vi "Calculate Waveform.vi"(6 "Channel":enum16{"Invalid", "Channel 1", "Channel 2"}(ring), 8 "error in (no error)":errorcluster, 9 "Acquisition Time":timestamp, 10 "Points":i16[](array[numeric]), 11 "OWON SDS1022 in":refnum<class "OWON SDS1022.lvclass">) -> (0 "error out":errorcluster, 3 "OWON SDS1022 out":refnum<class "OWON SDS1022.lvclass">)   [LabVIEW 2023, in "OWON SDS1022.lvclass"]
uses:
  Continuous Waveform Acq CFG.lvclass/Continuous Waveform Acq CFG.ctl
  OWON SDS1022.lvclass
  OWON SDS1022.lvclass/OWON SDS1022.ctl
  5ff70b4c-a951-438e-aa90-247ca6a210be.vi
  <vilib>/Utility/error.llb/Error Cluster From Error Code.vi
  <vilib>/ErrorRing/Error Ring.xnode
  f43ade27-b117-4f32-80ae-6d7f201a5a9d.vi
  7c31662c-ba05-4203-8e23-b7890d435081.vi
  b003ad20-f1c5-4d81-8556-46127c723614.vi
  HAL/Scope Base/Scope Base.lvclass
  E:/git/HAL/Scope VISA/Scope VISA.lvclass
  E:/git/HAL/Scope Base/Scope Base.lvclass
  E:/git/HAL/Hardware_class/Instrument.lvclass
  E:/git/HAL/Interfaces/IScope/IScope.lvclass
  E:/git/OWON-SDS1022-LabVIEW/OWON SDS1022/OWON SDS1022.lvclass
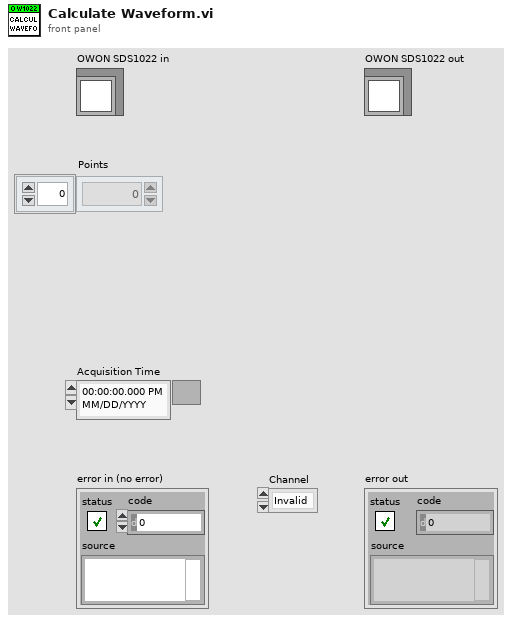
[diagram p1: front panel]
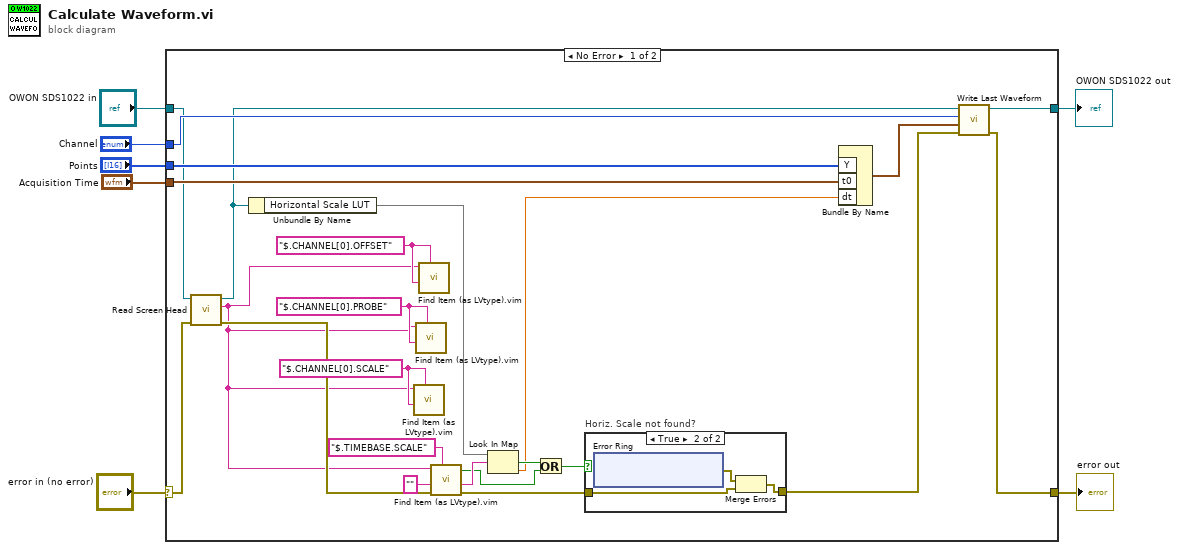
[diagram p0: block diagram]
diagram:
  n1 = case shown="No Error" "error in (no error)" {
    selector: "error in (no error)" -> [w27 w42]
    tunnel: [w14 w42] -> w6
    tunnel: [w13 w41] -> w4
    tunnel: "OWON SDS1022 in" -> [w10 w41]
    tunnel: "Points" -> [w23 _]
    tunnel: "Acquisition Time" -> [w22 _]
    tunnel: "Channel" -> [w12 _]
    frame No Error {
      w17 = "$.CHANNEL[0].OFFSET" ("$Path or Item Name")
      w16 = "$.CHANNEL[0].PROBE" ("$Path or Item Name")
      w15 = "$.CHANNEL[0].SCALE" ("$Path or Item Name")
      n2 = call "Read Screen Head.vi"("error in"=w27, "OWON SDS1022.lvclass"=w10) -> ("error out"=w30:errorcluster, "Head <JSON>"=w9:string, "OWON SDS1022.lvclass 2"=w8:refnum<class "OWON SDS1022.lvclass">)  [unwired: 7 in]
      n3 = Unbundle By Name(w8) -> ("Horizontal Scale LUT"=w19:map{string, dbl})
      n4 = call "Find Item (as LVtype).vim"("$Path or Item Name"=w15, "Data Type and Default Value"=w15, "JSON"=w9) -> ()  [unwired: 5 in, 4 out]
      n5 = call "Find Item (as LVtype).vim"("$Path or Item Name"=w16, "Data Type and Default Value"=w16, "JSON"=w9) -> ()  [unwired: 5 in, 4 out]
      n6 = call "Find Item (as LVtype).vim"("$Path or Item Name"=w17, "Data Type and Default Value"=w17, "JSON"=w9) -> ()  [unwired: 5 in, 4 out]
      n7 = call "Find Item (as LVtype).vim"("$Path or Item Name"="$.TIMEBASE.SCALE", "error in (no error)"=w30, "Data Type and Default Value"="", "JSON"=w9) -> ("error out"=w26:errorcluster, "Data"=w28:string, "Found"=w20:bool)  [unwired: 4 in, 1 out]
      n8 = Look In Map(map=w19, key=w28) -> (key not found?=w24:bool, value=w18:dbl)  [unwired: 1 in]
      n9 = Or(x=w24, y=w20) -> (x .or. y?=w21:bool)
      n10 = case "Horiz. Scale not found?" shown="True" w21 {
        tunnel: w26 -> [w32 w34]
        tunnel: [w32 w33] -> w25
        frame False {
        }
        frame True {
          n11 = xnode "Error Ring"() -> ("error out"=w35:errorcluster)
          n12 = Merge Errors(w35, w34) -> (w33:errorcluster)
        }
      }
      n13 = Bundle By Name("Y"=w23, "t0"=w22, "dt"=w18) -> (w11:waveform(i16))  [unwired: 1 in]
      n14 = call "Write Last Waveform.vi"("error in (no error)"=w25, "Last Waveform"=w11, "Channel"=w12, "Scope Base in"=w8) -> ("error out"=w14:errorcluster, "Scope Base out"=w13:refnum<class "OWON SDS1022.lvclass">)  [unwired: 6 in]
    }
    frame Error {
    }
  }
  "error out" <- w6
  "OWON SDS1022 out" <- w4
